vi "programa3.vi"() -> ()   [LabVIEW 2011]
panel:
  out "Observación":string
  out "Alarma":bool
  out "Velocidad":i32(knob) scale=0.0..180.0
  out "Termperatura":dbl(slide) scale=0.0..100.0
  # "Generar la temperatura entre 1-100 y la velocidad entre 1-180.\nCuando la velocidad sea mayor a 100 debemos de escribir\nvelocidad ALTA y cuando la temperatura sea mayor a 80 y la\n velocidad mayor a 120 se debe encender la alarma."
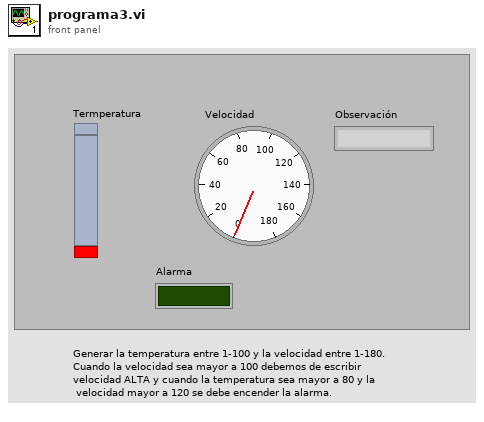
[diagram p1: front panel]
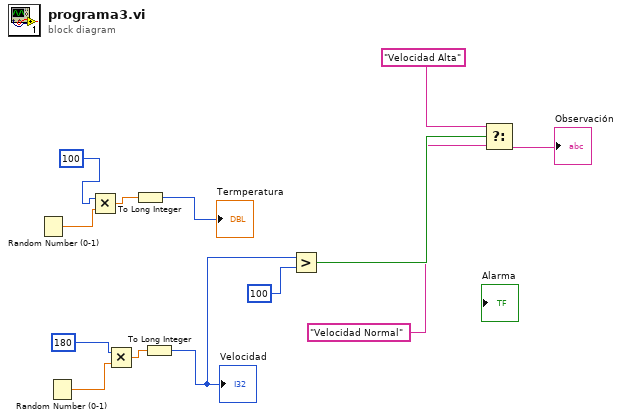
[diagram p0: block diagram]
diagram:
  n1 = Random Number (0-1)() -> (number: 0 to 1=w11:dbl)
  n2 = Random Number (0-1)() -> (number: 0 to 1=w10:dbl)
  n3 = Multiply(x=100, y=w11) -> (x*y=w9:dbl)
  n4 = Multiply(x=180, y=w10) -> (x*y=w8:dbl)
  n5 = To Long Integer(number=w9) -> (32bit integer=→"Termperatura":i32)
  n6 = To Long Integer(number=w8) -> (32bit integer=w6:i32)
  "Velocidad" <- w6
  n7 = Greater?(x=w6, y=100) -> (0:w3:bool)
  n8 = Select(t="Velocidad Alta", s=w3, f="Velocidad Normal") -> (s? t:f=→"Observación":string)
